vi "niRFUtil MASMT Resample (constant to constant)_Resample (CSG).vi"(4 "max decimation":i32=1000, 6 "Resample FIR":sgl[](array[numeric]), 7 "reset?":bool, 8 "error in (no error)":errorcluster, 9 "config":T1 {"timing jitter" items=["Interpolation", "Rounding"]}, 10 "anti-aliasing?":bool=TRUE, 11 "X":csg[](array[numeric])) -> (0 "error out":errorcluster, 2 "t0":sgl, 3 "Y":csg[](array[numeric]))   [LabVIEW 2015, in "niRFUtil.lvlib"]
uses:
  niRFUtil.lvlib
  Utilities/niRFMASMT_FFT.dll
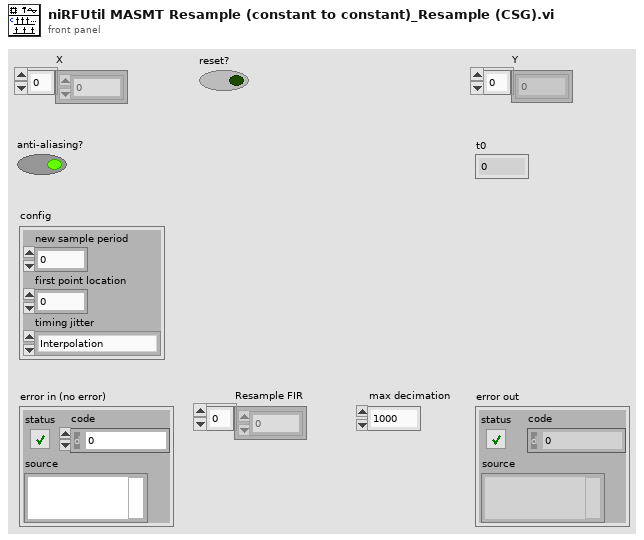
[diagram p1: front panel]
types:
  T1 = cluster{"new sample period":sgl, "first point location":sgl, "timing jitter":i32}
  T2 = cluster{"preConditionLen":i32, "extractFilterLeftLen":i32, "extractFilterRightLen":i32, "extractFilterMethod":i32, "extractFilterScaling":dbl, "samplingPeriod":dbl, "startTime":dbl, "offset":dbl, "index":i32}
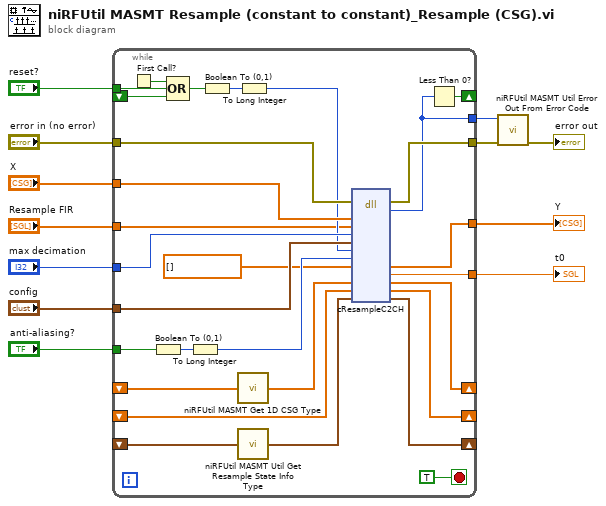
[diagram p0: block diagram]
diagram:
  n1 = while {
    tunnel: "X" -> [w41]
    tunnel: "config" -> [w40]
    tunnel: "error in (no error)" -> [w39]
    tunnel: [w38] -> w1
    tunnel: "anti-aliasing?" -> [w37]
    tunnel: "Resample FIR" -> [w16]
    tunnel: "max decimation" -> [w35]
    tunnel: [w24] -> w11
    tunnel: [w33] -> w12
    tunnel: [w32] -> w2
    tunnel: "reset?" -> [w22]
    shift-right: [w29] -> _
    shift-left: _ -> [w15]
    shift-right: [w30] -> _
    shift-left: _ -> [w26]
    shift-right: [w23] -> _
    shift-left: _ -> [w21]
    shift-right: [w28] -> _
    shift-left: _ -> [w17]
    stop <- TRUE stop-if-true
    n2 = First Call?() -> (First Call?: T/F=w18:bool)
    n3 = Boolean To (0,1)(Boolean=w37) -> (0, 1=w36:i16)
    n4 = Compound Arithmetic op=OR(w18, w22, w21) -> (w19:bool)
    n5 = To Long Integer(number=w36) -> (32bit integer=w34:i32)
    n6 = Boolean To (0,1)(Boolean=w19) -> (0, 1=w20:i16)
    n7 = call "niRFUtil MASMT Get 1D CSG Type.vi"("1D CSG Array in"=w15) -> ("1D CSG Array out"=w14:csg[])
    n8 = call "niRFUtil MASMT Util Get Resample State Info Type.vi"("resample state info in"=w26) -> ("resample state info out"=w25:T2)
    n9 = To Long Integer(number=w20) -> (32bit integer=w31:i32)
    n10 = dll-call lib="C:/Perforce/semoore-sales/Customers/NATI-3813/Noise Floor/LV Filters/ParallelComplexFilterRFUtil/niRFUtil/MASMT/Utilities/niRFMASMT_FFT.*" fn="cResampleC2CH"(error in=w39, "xH"=w41, "pfilterCoefH"=w16, "pfilterMaxDecimation"=w35, "config"=w40, "reset"=w31, "bandLimit"=w34, "yH"=csg[] [], "xBufferH"=w14, "extractFilterH"=w17, "state"=w25) -> (error out=w33:errorcluster, "error"=w24:i32, "yH"=w32:csg[], "t0"=w38:sgl, "xBufferH"=w29:csg[], "extractFilterH"=w28:sgl[], "state"=w30:T2)  [unwired: 9 in, 1 out]
    n11 = Less Than 0?(x=w24) -> (x < 0?=w23:bool)
  }
  "t0" <- w1
  "Y" <- w2
  n12 = call "niRFUtil MASMT Util Error Out From Error Code.vi"("error in (no error)"=w12, "error code"=w11) -> ("error out"=→"error out":errorcluster)  [unwired: 9 in]
